vi "setup_process_queues.vi"(11 "Tool Assignments":T1) -> (0 "Process queue names out":string[](array[string]), 3 "Process queues":refnum<queue>[](array[refnum]))   [LabVIEW 2017, in "labview-standard-library.lvlib" / "automode-scripting.lvlib"]
uses:
  automode-scripting.lvlib
  type-defs/command_line_info.ctl
  type-defs/tool-assignments.ctl
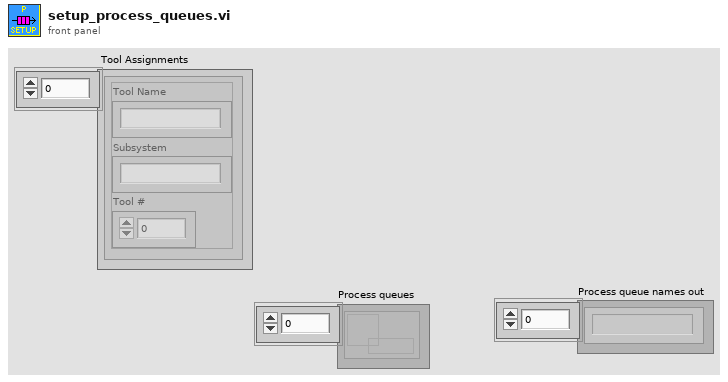
[diagram p1: front panel]
types:
  T1 = typedef "tool-assignments.ctl" = cluster{"Tool Name":string, "Subsystem":string, "Tool #":i32}[]
  T2 = typedef "labview-standard-library.lvlib/automode-scripting.lvlib/command_line_info.ctl" = cluster{"Line text":string, "Line #":i32}
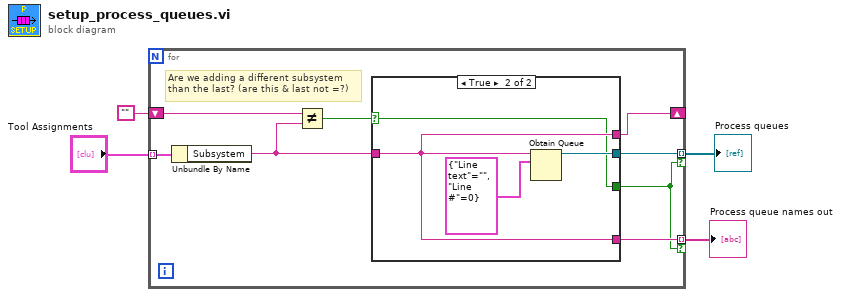
[diagram p0: block diagram]
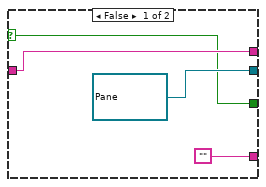
[diagram p2: hidden frame]
diagram:
  n1 = for {
    tunnel: "Tool Assignments" -> [w11] mode=indexing
    tunnel: [w12] -> w4 mode=indexing if=w5
    tunnel: [w9] -> w2 mode=indexing if=w5
    shift-right: [w6] -> _
    shift-left: "" -> [w10]
    # "Are we adding a different subsystem\nthan the last? (are this & last not =?)"
    n2 = Unbundle By Name(w11) -> ("Subsystem"=w7:string)
    n3 = Not Equal?(x=w10, y=w7) -> (x != y?=w8:bool)
    n4 = case shown="True" w8 {
      selector: w8 -> [w13 w17]
      tunnel: [refnum<queue> refnum ("queue out") w20] -> w12
      tunnel: w7 -> [w15 w18]
      tunnel: ["" w18] -> w9
      tunnel: [w15 w18] -> w6
      tunnel: [w13 w17] -> w5
      frame False {
      }
      frame True {
        n5 = Obtain Queue(name (unnamed)=w18, element data type=T2 {"Line text"="", "Line #"=0}) -> (queue out=w20:refnum<queue>)  [unwired: 3 in, 2 out]
      }
    }
  }
  "Process queues" <- w4
  "Process queue names out" <- w2
